vi "CST_1299ShadowRegister.VI"() -> (1 "DUTRegisters":T2={"ID"={"REV_ID"=0, "DEV_ID"=0}, "Config1 "={"DAISY_EN"=enum."Daisy Chain Mode", "CLK_EN"=enum."Output Disabled", "DR"=enum."f(MOD) /64"}, "Config2 "={"INT_CAL"=enum."Driven Externally", "CAL_AMP"=enum."(VREFP-VREFN)/2.4", "CAL_FREQ"=enum."f(CLK)/2^21"}, "Config3 "={"PD_REFBUF"=enum."Disabled", "BIAS_MEAS"=enum."Open", "BIASREF_INT"=enum."BIASREF fed externally", "PD_BIAS"=enum."Disabled"}, "Config4"={"PD_LOFF_COMP"=enum."Comparator Disabled"}, "CH1SET"={"PD#"=enum."Normal Operation", "GAIN#"=enum."6", "SRB2"=enum."Open (Off)", "MUX#"=enum."Normal Electrode"}, "CH2SET"={"PD#"=enum."Normal Operation", "GAIN#"=enum."6", "SRB2"=enum."Open (Off)", "MUX#"=enum."Normal Electrode"}, "CH3SET"={"PD#"=enum."Normal Operation", "GAIN#"=enum."6", "SRB2"=enum."Open (Off)", "MUX#"=enum."Normal Electrode"}, "CH4SET"={"PD#"=enum."Normal Operation", "GAIN#"=enum."6", "SRB2"=enum."Open (Off)", "MUX#"=enum."Normal Electrode"}, "CH5SET"={"PD#"=enum."Normal Operation", "GAIN#"=enum."6", "SRB2"=enum."Open (Off)", "MUX#"=enum."Normal Electrode"}, "CH6SET"={"PD#"=enum."Normal Operation", "GAIN#"=enum."6", "SRB2"=enum."Open (Off)", "MUX#"=enum."Normal Electrode"}, "CH7SET"={"PD#"=enum."Power-down", "GAIN#"=enum."6", "SRB2"=enum."Open (Off)", "MUX#"=enum."Normal Electrode"}, "CH8SET"={"PD#"=enum."Normal Operation", "GAIN#"=enum."6", "SRB2"=enum."Open (Off)", "MUX#"=enum."Normal Electrode"}, "MISC2"={"RegValue"=0.0}, "MISC1"={"SRB1"=enum."Open (Off)"}, "LOFF "={"COMP_TH"=enum."Positive - 90% : Negative - 10%", "ILEAD_OFF"=enum."6nA", "FLEAD_OFF"=enum."AC lead-off detection at SYS_CLK/(2^18)"}, "BIASSENSP"=[], "BIASSENSN"=[], "LOFF_STATP"=[], "LOFF_STATN"=[], "LOFF_SENSP"=[], "LOFF_SENSN"=[], "LOFF_FLIP"=[], "GPIO"={"Data"=[], "Direction"=[]}} {"ID"."DEV_ID" items=["ADS1294", "ADS1296", "ADS1298", "N/A", "ADS1194", "ADS1196", "ADS1198"]}, 2 "ShadowReg Reg Refs":T1)   [LabVIEW 2010]
doc: "This VI is a constant for the shadow register to store values during app.\n\nInputs:\n<None>\n\nOutputs:\nDUTRegisters (typedef of cooresponding control)\nShadowReg Reg Refs - (cluster[]) names and references to the controls in the shadow register. Allows for searching and indexing."
uses:
  Controls/Shift Registers/TYP_1299ShadowRegister.ctl
  Controls/Register/TYP_Reg_ID.ctl
  Controls/Register/TYP_Reg_CONFIG1.ctl
  Controls/Register/TYP_Reg_CONFIG2.ctl
  Controls/Register/TYP_Reg_CONFIG3.ctl
  Controls/Register/TYP_Reg_CONFIG4.ctl
  Controls/Register/TYP_Reg_CHxSET.ctl
  Controls/Register/TYP_Reg_MISC2.ctl
  Controls/Register/TYP_Reg_MISC1.ctl
  Controls/Register/TYP_Reg_LOFF.ctl
  Controls/Shift Registers/TYP_CtrlNameArray.ctl
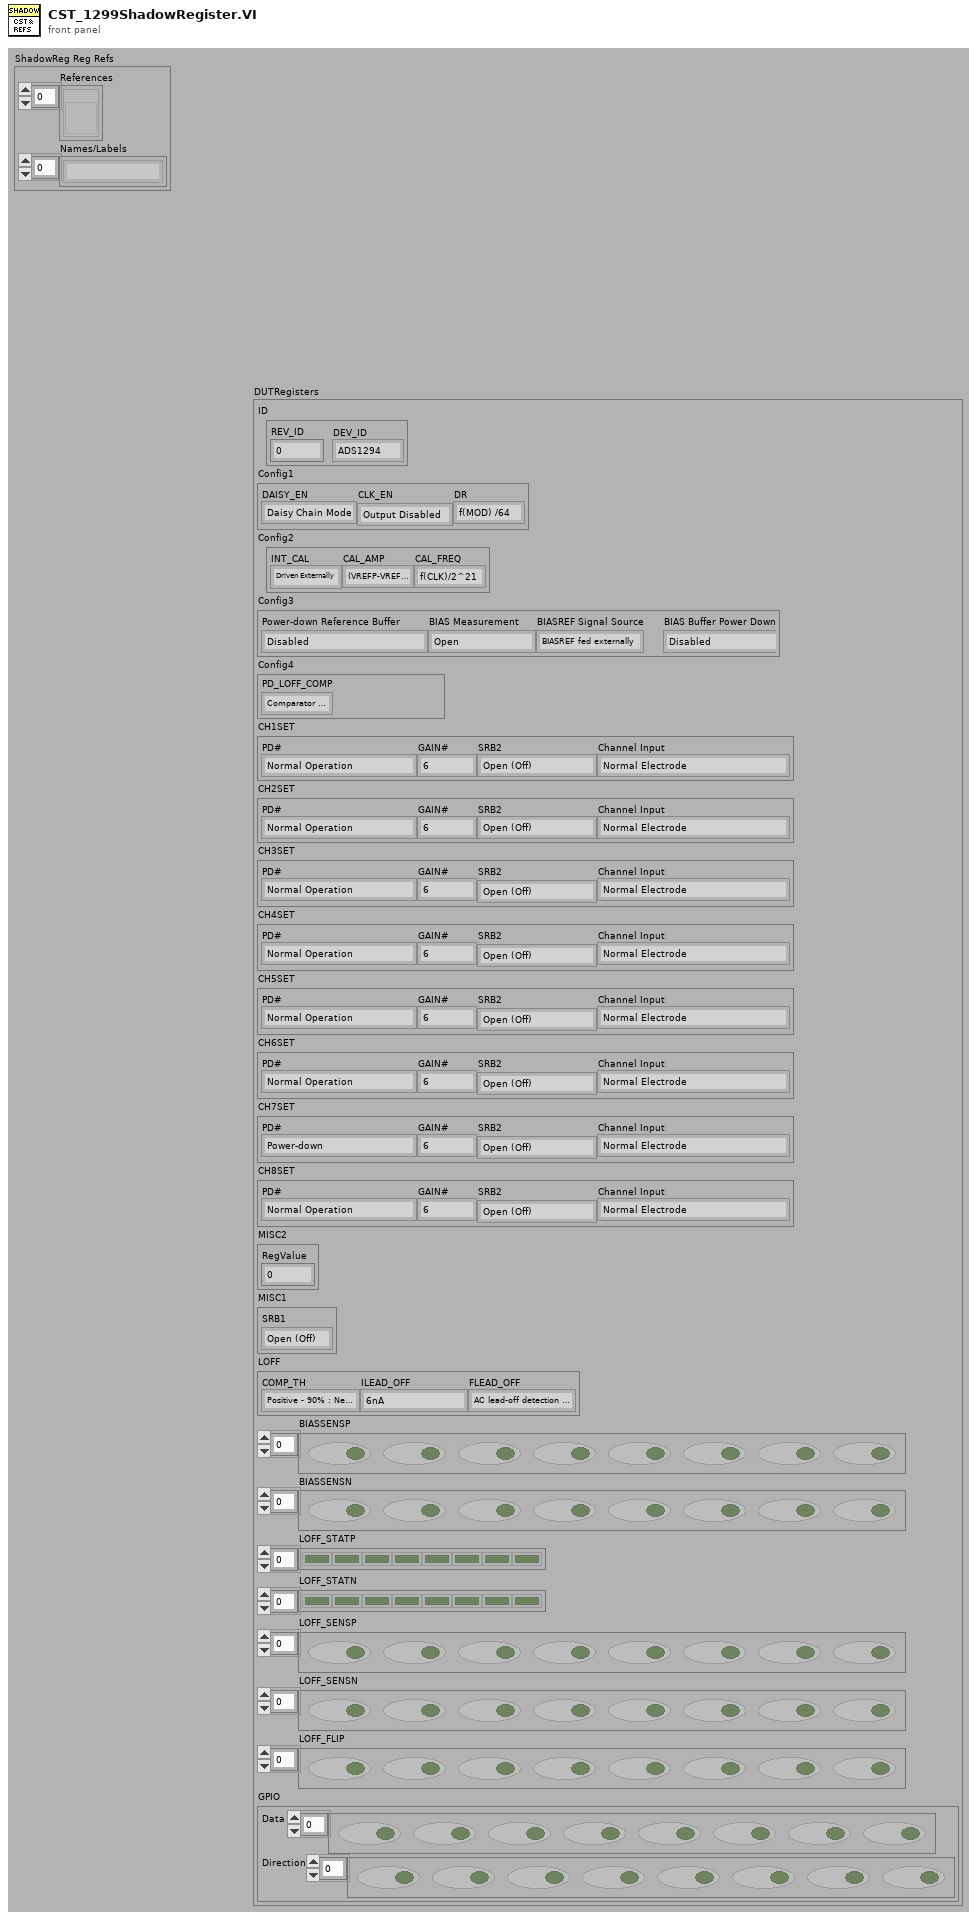
[diagram p1: front panel]
types:
  T1 = typedef "TYP_CtrlNameArray.ctl" = cluster{"References":refnum<vi>[], "Names/Labels":string[]}
  T2 = typedef "TYP_1299ShadowRegister.ctl" = cluster{"ID":T3, "Config1 ":T4, "Config2 ":T5, "Config3 ":T6, "Config4":T7, "CH1SET":T8, "CH2SET":T8, "CH3SET":T8, "CH4SET":T8, "CH5SET":T8, "CH6SET":T8, "CH7SET":T8, "CH8SET":T8, "MISC2":T9, "MISC1":T10, "LOFF ":T11, "BIASSENSP":bool[], "BIASSENSN":bool[], "LOFF_STATP":bool[], "LOFF_STATN":bool[], "LOFF_SENSP":bool[], "LOFF_SENSN":bool[], "LOFF_FLIP":bool[], "GPIO":cluster{"Data":bool[], "Direction":bool[]}}
  T3 = typedef "TYP_Reg_ID.ctl" = cluster{"REV_ID":u8, "DEV_ID":u16}
  T4 = typedef "TYP_Reg_CONFIG1.ctl" = cluster{"DAISY_EN":enum16{"Daisy Chain Mode", "Multiple Readback Mode"}, "CLK_EN":enum16{"Output Disabled", "Output Enabled"}, "DR":enum16{"f(MOD) /64", "f(MOD) /128", "f(MOD) /256", "f(MOD) /512", "f(MOD) /1024", "f(MOD) /2048", "f(MOD) /4096"}}
  T5 = typedef "TYP_Reg_CONFIG2.ctl" = cluster{"INT_CAL":enum16{"Driven Externally", "Generated Internally"}, "CAL_AMP":enum16{"(VREFP-VREFN)/2.4", "2x(VREFP-VREFN)/2.4"}, "CAL_FREQ":enum16{"f(CLK)/2^21", "f(CLK)/2^20", "N/A", "DC"}}
  T6 = typedef "TYP_Reg_CONFIG3.ctl" = cluster{"PD_REFBUF":enum16{"Disabled", "Enabled"}, "BIAS_MEAS":enum16{"Open", "BIASIN Routed"}, "BIASREF_INT":enum16{"BIASREF fed externally", "BIASREF = (AVDD-AVSS)/2"}, "PD_BIAS":enum16{"Disabled", "Enabled"}}
  T7 = typedef "TYP_Reg_CONFIG4.ctl" = cluster{"PD_LOFF_COMP":enum16{"Comparator Disabled", "Comparator Enabled"}}
  T8 = typedef "TYP_Reg_CHxSET.ctl" = cluster{"PD#":enum16{"Normal Operation", "Power-down"}, "GAIN#":enum16{"1", "2", "4", "6", "8", "12", "24"}, "SRB2":enum16{"Open (Off)", "Closed (On)"}, "MUX#":enum16{"Normal Electrode", "Input Short", "BIAS Measurement", "MVDD", "Temperature Sensor", "Test Signal", "BIAS Positive Electrode Driver", "BIAS Negative Electrode Driver"}}
  T9 = typedef "TYP_Reg_MISC2.ctl" = cluster{"RegValue":dbl}
  T10 = typedef "TYP_Reg_MISC1.ctl" = cluster{"SRB1":enum16{"Open (Off)", "Closed (On)"}}
  T11 = typedef "TYP_Reg_LOFF.ctl" = cluster{"COMP_TH":enum16{"Positive - 95% : Negative - 5%", "Positive - 92.5% : Negative - 7.5%", "Positive - 90% : Negative - 10%", "Positive - 87.5% : Negative - 12.5%", "Positive - 85% : Negative - 15%", "Positive - 80% : Negative - 20%", "Positive - 75% : Negative - 25%", "Positive - 70% : Negative - 30%"}, "ILEAD_OFF":enum16{"6nA", "24nA", "6uA", "24uA"}, "FLEAD_OFF":enum16{"DC lead-off detection", "AC lead-off detection at SYS_CLK/(2^18)", "AC lead-off detection at SYS_CLK/(2^16)", "AC lead-off detection at fdr/4"}}
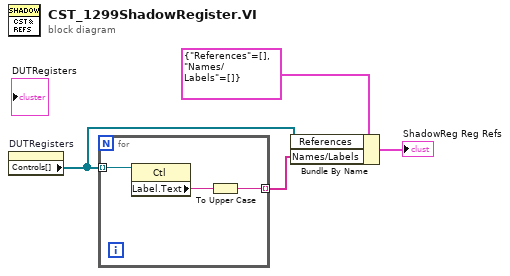
[diagram p0: block diagram]
diagram:
  n1 = property on="DUTRegisters" class="Clust (strict)"() -> ("Controls[]"=w4:refnum<vi>[])  [unwired: 2 in, 2 out]
  n2 = for {
    tunnel: w4 -> [w7] mode=indexing
    tunnel: [w5] -> w3 mode=indexing
    n3 = property class="Ctl"(reference=w7) -> ("Label.Text"=w6:string)  [unwired: 1 in, 2 out]
    n4 = To Upper Case(1:w6) -> (0:w5:string)
  }
  n5 = Bundle By Name(cluster=T1 {"References"=[], "Names/Labels"=[]} ("ControlRef Array"), "References"=w4, "Names/Labels"=w3) -> (→"ShadowReg Reg Refs":T1)
